vi "DatabaseWriter.vi"() -> ()   [LabVIEW 2023]
panel:
  out "Location of DAQ":string
  in  "On/Off":bool
  out "On/Off Light":bool
  in  "Exit":bool
  out "Data Chart":dbl(graph)
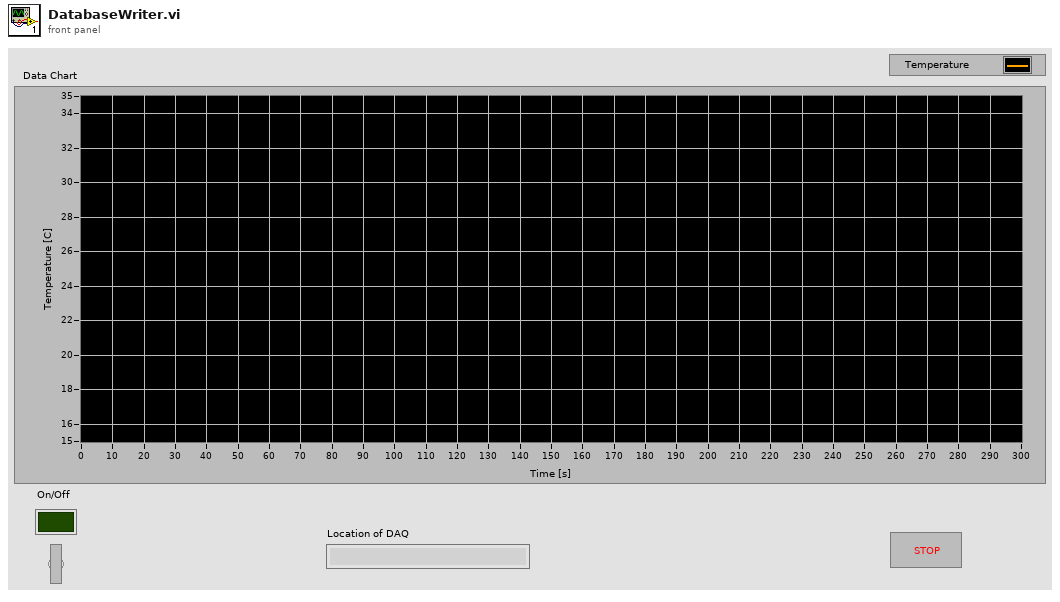
[diagram p1: front panel]
types:
  T1 = typedef "NI_Database_API.lvlib/Conn ObjectReference.ctl" = refnum<k1>
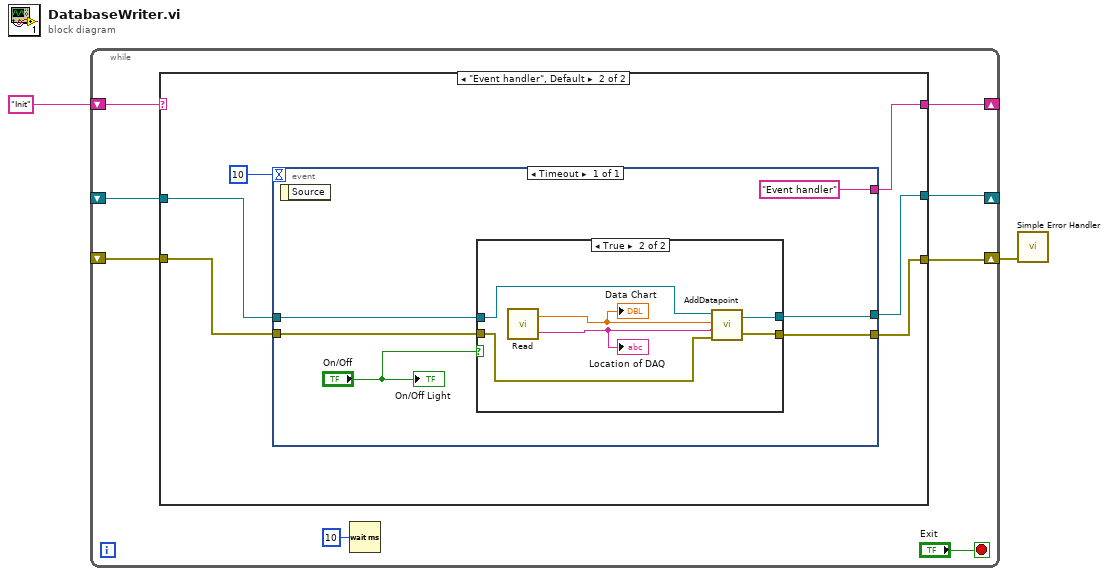
[diagram p0: block diagram]
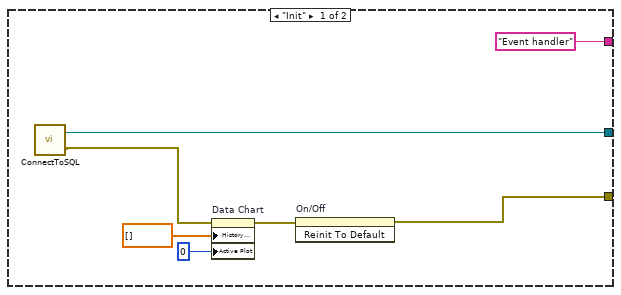
[diagram p2: hidden frame]
diagram:
  n1 = while {
    shift-right: [w8] -> _
    shift-left: "Init" -> [w9]
    shift-right: [w7] -> _
    shift-left: _ -> [w4]
    shift-right: [w6] -> w1
    shift-left: _ -> [w5]
    stop <- "Exit" stop-if-true
    n2 = case shown="\"Event handler\", Default" w9 {
      tunnel: [w11 w18] -> w6
      tunnel: ["Event handler" w22] -> w8
      tunnel: [w14 w19] -> w7
      tunnel: w5 -> [_ w20]
      tunnel: w4 -> [_ w21]
      frame "Init" {
        n3 = call "ConnectToSQL.vi"() -> ("error out"=w13:errorcluster, "connection reference"=w14:T1)  [unwired: 2 in]
        n4 = property on="Data Chart" class="WFChart (strict)"(error in=w13, "History Data"=dbl[] [], "Active Plot"=u32 0) -> (error out=w12:errorcluster)  [unwired: 1 in, 1 out]
        n5 = invoke on="On/Off" class="Bool (strict)" method="Reinit To Default"(error in=w12) -> (error out=w11:errorcluster)  [unwired: 2 in, 2 out]
      }
      frame "Event handler", Default {
        n6 = event shown="[0] Timeout" {
          selector: _ -> [_]
          dyn-events: _ -> [_]
          timeout: 10 -> [_]
          tunnel: ["Event handler"] -> w22
          tunnel: w21 -> [w28]
          tunnel: w20 -> [w27]
          tunnel: [w26] -> w19
          tunnel: [w25] -> w18
          event Timeout {
            n7 = event-data() -> ()  [unwired: 1 in, 1 out]
            n8 = case shown="True" "On/Off" {
              tunnel: w28 -> [w30 w37]
              tunnel: w27 -> [w31 w36]
              tunnel: [w30 w34] -> w26
              tunnel: [w31 w35] -> w25
              frame False {
              }
              frame True {
                n9 = call "Read.vi"() -> ("Read Number"=w33:dbl, "Read Location"=w32:string)  [unwired: 1 in]
                "Data Chart" <- w33
                "Location of DAQ" <- w32
                n10 = call "AddDatapoint.vi"("error in (no error)"=w36, "Location of DAQ"=w32, "Temperature In"=w33, "connection reference in"=w37) -> ("error out"=w35:errorcluster, "connection reference out"=w34:T1)
              }
            }
            "On/Off Light" <- "On/Off"
          }
        }
      }
    }
    n11 = Wait (ms)(milliseconds to wait=u32 10) -> ()  [unwired: 1 out]
  }
  n12 = call <vilib>:"Simple Error Handler.vi"("error in (no error)"=w1) -> ()  [unwired: 4 in, 5 out]
